vi "Frame Multiple.vi"() -> ()   [LabVIEW 2021]
uses:
  <userlib>/SciSDK/SciSDK_Labview.lvlib
panel:
  out "Frame Buffer Out":T1
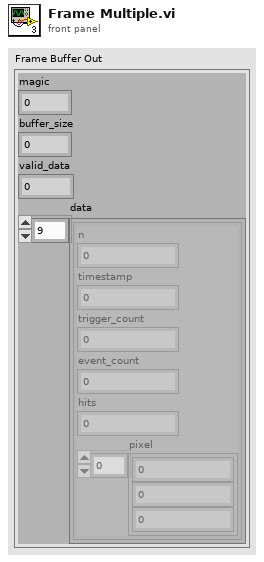
[diagram p1: front panel]
types:
  T1 = cluster{"magic":u32, "buffer_size":u32, "valid_data":u32, "data":cluster{"n":u64, "timestamp":u64, "trigger_count":u64, "event_count":u64, "hits":u64, "pixel":u32[]}[]}
  T2 = cluster{"Name":string, "Board Model":string, "Handle":u64}
  T3 = cluster{"Frame Path":string, "Frame Name":string}
  T4 = cluster{"Board Name":string, "Board Model":string, "Handle":u64}
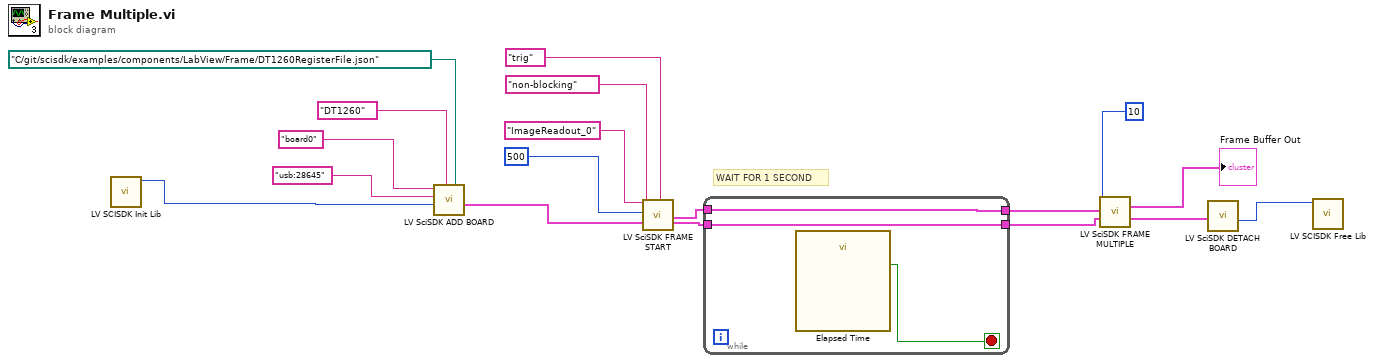
[diagram p0: block diagram]
diagram:
  # "WAIT FOR 1 SECOND"
  n1 = call <userlib>:"LV SCISDK Init Lib.vi"() -> ("function return"=w14:u64)  [unwired: 11 in]
  n2 = call <userlib>:"LV SciSDK ADD BOARD.vi"("JsonFile"=path "C:/git/scisdk/examples/components/LabView/Frame/DT1260RegisterFile.json", "Board Model"="DT1260", "SciSDK Handle"=w14, "DevicePath"="usb:28645", "Name"="board0") -> ("Board Handle Out"=w12:T2)  [unwired: 4 in, 2 out]
  n3 = call <userlib>:"LV SciSDK FRAME START.vi"("Frame Name"="ImageReadout_0", "Acq Mode"="non-blocking", "Timeout"=500, "Board Handle In"=w12, "Trigger Mode"="trig") -> ("Frame Handle Out"=w7:T3, "Board Handle Out"=w6:T4)  [unwired: 12 in, 1 out]
  n4 = while {
    tunnel: w7 -> [w20]
    tunnel: w6 -> [w19]
    tunnel: [w20] -> w5
    tunnel: [w19] -> w4
    stop <- w21 stop-if-true
    n5 = call "Elapsed Time"() -> ("Time has Elapsed"=w21:bool)  [unwired: 12 in, 7 out]
  }
  n6 = call <userlib>:"LV SciSDK FRAME MULTIPLE.vi"("Buffer Size"=10, "Frame Handle In"=w5, "Board Handle In"=w4) -> ("Frame Buffer Out"=→"Frame Buffer Out":T1, "Board Handle Out"=w1:T4)  [unwired: 8 in, 3 out]
  n7 = call <userlib>:"LV SciSDK DETACH BOARD.vi"("Board Handle In"=w1) -> ("SciSDK Handle"=w2:u64)  [unwired: 9 in, 1 out]
  n8 = call <userlib>:"LV SCISDK Free Lib.vi"("handle"=w2) -> ()  [unwired: 9 in, 2 out]
